vi "5) Target Groups.vi"() -> ()   [LabVIEW 2020, in "VectoScratch.lvlib"]
uses:
  VectoScratch.lvlib
  Vecto/Connection State.ctl
  Vecto/proto/TcpClientHello/Data.ctl
  Simple TCP Handler/Simple TCP Handler.lvclass
  C:/dev/lv20CE/relink/lv-vecto/Vecto/TCPConnectionHandler/TCPConnectionHandler.lvclass
  C:/dev/lv20CE/relink/lv-vecto/Vecto/TCPMessageHandler/TCPMessageHandler.lvclass
  Vecto/TCPMessaging/TCPMessaging.lvclass
  Vecto/TCPMessageService/TCPMessageAPI.lvclass
  Vecto/proto/TcpClientHello/TcpClientHello.lvlib
  Vecto/SequenceCountService/SequenceCountService.lvclass
  Vecto/Vecto.lvlib
panel:
  in  "Stop 3":bool
  in  "Target 3":u32=5
  in  "Target 2":u32=7
  in  "Target 1":u32=6
  in  "Groups":cluster{"Targets":u32[]}[](array[cluster])=[{"Targets"=[4, 5, 7]}, {"Targets"=[4, 5, 6]}, {"Targets"=[4, 6, 7]}]
  in  "Send 3":bool
  out "Read 3":i32
  in  "Send 2":bool
  out "Read 2":i32
  in  "Send 1":bool
  out "Read 1":i32
  out "Error 2":errorcluster
  in  "Stop 2":bool
  out "State 2":T1=enum."Disconnected"
  out "Server Error":errorcluster
  out "Error 1":errorcluster
  in  "Stop 1":bool
  out "State 3":T1=enum."Disconnected"
  out "State 1":T1=enum."Disconnected"
  # "Each node (Clients 1 & 2, Server 3) should also receive data for the targets configured below.\n\nEach row is each of the nodes in order."
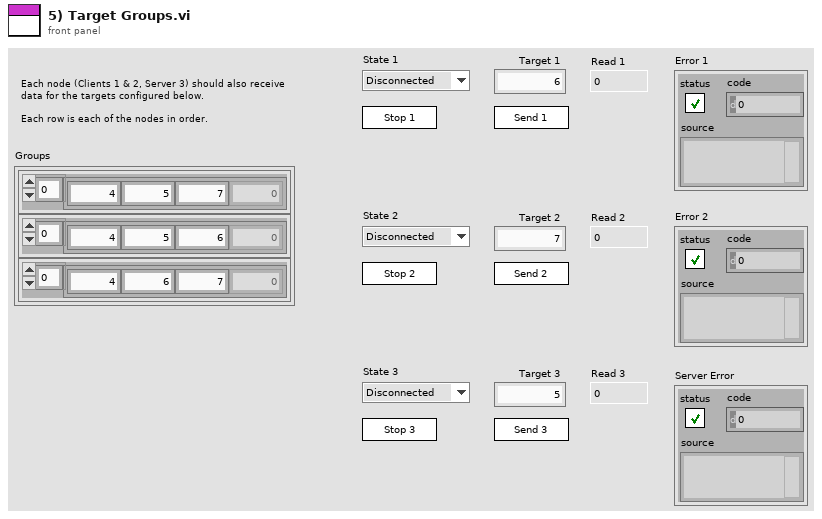
[diagram p1: front panel]
types:
  T1 = typedef "Vecto.lvlib/Connection State.ctl" = enum16{"Connected", "Disconnected"}
  T2 = typedef "TcpClientHello.lvlib/Data.ctl" = cluster{"node_id":u32, "system":string, "cluster":string, "node_name":string, "app_version":string, "config_version":string}
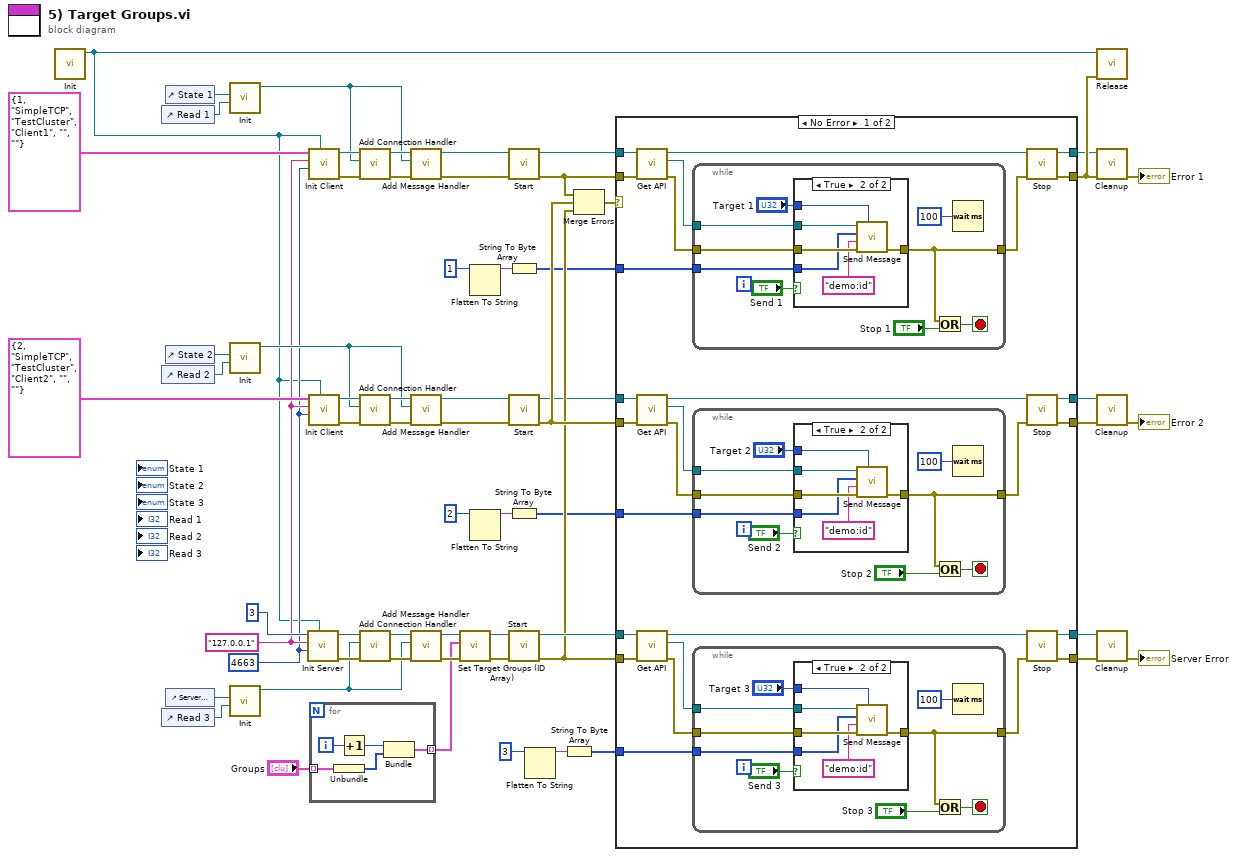
[diagram p0: block diagram]
diagram:
  w2 = u16 4663 ("Bind Port")
  w3 = "127.0.0.1" ("Bind Address")
  n1 = call "Init.vi"() -> ("SequenceCountService out"=w1:refnum<class "SequenceCountService.lvclass">)  [unwired: 10 in, 1 out]
  n2 = control-ref of="Read 1"() -> (w25:refnum<vi>)
  n3 = control-ref of="Read 2"() -> (w24:refnum<vi>)
  n4 = control-ref of="Read 3"() -> (w17:refnum<vi>)
  n5 = control-ref of="State 1"() -> (w59:refnum<vi>)
  n6 = control-ref of="State 2"() -> (w26:refnum<vi>)
  n7 = control-ref of="Server State"() -> (w51:refnum<vi>)
  n8 = call "Init.vi"("Value"=w25, "State"=w59) -> ("Simple TCP Handler out"=w55:refnum<class "Simple TCP Handler.lvclass">)  [unwired: 8 in, 1 out]
  n9 = call "Init.vi"("Value"=w24, "State"=w26) -> ("Simple TCP Handler out"=w23:refnum<class "Simple TCP Handler.lvclass">)  [unwired: 8 in, 1 out]
  n10 = call "Init.vi"("Value"=w17, "State"=w51) -> ("Simple TCP Handler out"=w36:refnum<class "Simple TCP Handler.lvclass">)  [unwired: 8 in, 1 out]
  n11 = call "Init Server.vi"("SequenceCountService"=w1, "Bind Port"=w2, "Bind Address"=w3, "Node ID"=u32 3) -> ("error out"=w46:errorcluster, "TCPMessaging out"=w47:refnum<class "TCPMessaging.lvclass">)  [unwired: 6 in]
  n12 = call "Init Client.vi"("SequenceCountService"=w1, "Remote Port"=w2, "Remote Address"=w3, "Client Info"=T2 {"node_id"=1, "system"="SimpleTCP", "cluster"="TestCluster", "node_name"="Client1", "app_version"="", "config_version"=""}) -> ("error out"=w57:errorcluster, "TCPMessaging out"=w58:refnum<class "TCPMessaging.lvclass">)  [unwired: 6 in]
  n13 = call "Init Client.vi"("SequenceCountService"=w1, "Remote Port"=w2, "Remote Address"=w3, "Client Info"=T2 {"node_id"=2, "system"="SimpleTCP", "cluster"="TestCluster", "node_name"="Client2", "app_version"="", "config_version"=""}) -> ("error out"=w28:errorcluster, "TCPMessaging out"=w27:refnum<class "TCPMessaging.lvclass">)  [unwired: 6 in]
  n14 = for {
    tunnel: "Groups" -> [w66] mode=indexing
    tunnel: [w63] -> w18 mode=indexing
    i -> [w67]
    n15 = Unbundle(w66) -> ("Targets"=w64:u32[])
    n16 = Increment(x=w67) -> (x+1=w65:i32)
    n17 = Bundle(w65, "Targets"=w64) -> (w63:cluster{i32, "Targets":u32[]})  [unwired: 1 in]
  }
  n18 = call "Add Connection Handler.vi"("error in (no error)"=w57, "TCPConnectionHandler"=w55, "TCPMessaging in"=w58) -> ("error out"=w54:errorcluster, "TCPMessaging out"=w56:refnum<class "TCPMessaging.lvclass">)  [unwired: 7 in]
  n19 = call "Add Connection Handler.vi"("error in (no error)"=w28, "TCPConnectionHandler"=w23, "TCPMessaging in"=w27) -> ("error out"=w30:errorcluster, "TCPMessaging out"=w29:refnum<class "TCPMessaging.lvclass">)  [unwired: 7 in]
  n20 = call "Add Connection Handler.vi"("error in (no error)"=w46, "TCPConnectionHandler"=w36, "TCPMessaging in"=w47) -> ("error out"=w49:errorcluster, "TCPMessaging out"=w48:refnum<class "TCPMessaging.lvclass">)  [unwired: 7 in]
  n21 = call "Add Message Handler.vi"("error in (no error)"=w54, "TCPMessageHandler"=w55, "TCPMessaging in"=w56) -> ("error out"=w52:errorcluster, "TCPMessaging out"=w53:refnum<class "TCPMessaging.lvclass">)  [unwired: 7 in]
  n22 = call "Add Message Handler.vi"("error in (no error)"=w30, "TCPMessageHandler"=w23, "TCPMessaging in"=w29) -> ("error out"=w32:errorcluster, "TCPMessaging out"=w31:refnum<class "TCPMessaging.lvclass">)  [unwired: 7 in]
  n23 = call "Add Message Handler.vi"("error in (no error)"=w49, "TCPMessageHandler"=w36, "TCPMessaging in"=w48) -> ("error out"=w50:errorcluster, "TCPMessaging out"=w20:refnum<class "TCPMessaging.lvclass">)  [unwired: 7 in]
  n24 = call "Set Target Groups (ID Array).vi"("error in (no error)"=w50, "Target Groups"=w18, "TCPMessaging in"=w20) -> ("error out"=w21:errorcluster, "TCPMessaging out"=w19:refnum<class "TCPMessaging.lvclass">)  [unwired: 7 in]
  n25 = Flatten To String(anything=1) -> (data string=w12:string)  [unwired: 3 in, 2 out]
  n26 = Flatten To String(anything=2) -> (data string=w7:string)  [unwired: 3 in, 2 out]
  n27 = call "Start.vi"("error in (no error)"=w52, "TCPMessaging in"=w53) -> ("error out"=w44:errorcluster, "TCPMessaging out"=w42:refnum<class "TCPMessaging.lvclass">)  [unwired: 8 in]
  n28 = String To Byte Array(string=w12) -> (unsigned byte array=w10:u8[])
  n29 = call "Start.vi"("error in (no error)"=w32, "TCPMessaging in"=w31) -> ("error out"=w62:errorcluster, "TCPMessaging out"=w16:refnum<class "TCPMessaging.lvclass">)  [unwired: 8 in]
  n30 = String To Byte Array(string=w7) -> (unsigned byte array=w9:u8[])
  n31 = call "Start.vi"("error in (no error)"=w21, "TCPMessaging in"=w19) -> ("error out"=w34:errorcluster, "TCPMessaging out"=w43:refnum<class "TCPMessaging.lvclass">)  [unwired: 8 in]
  n32 = Flatten To String(anything=3) -> (data string=w6:string)  [unwired: 3 in, 2 out]
  n33 = String To Byte Array(string=w6) -> (unsigned byte array=w4:u8[])
  n34 = Merge Errors(w44, w62, w34) -> (w45:errorcluster)
  n35 = case shown="No Error" w45 {
    tunnel: w44 -> [w93 w148]
    tunnel: w34 -> [w91 w147]
    tunnel: w43 -> [w92 w146]
    tunnel: w42 -> [w94 w145]
    tunnel: [w82 w148] -> w61
    tunnel: [w84 w147] -> w39
    tunnel: [w85 w146] -> w40
    tunnel: [w86 w145] -> w41
    tunnel: w16 -> [w76 w144]
    tunnel: w62 -> [w74 w143]
    tunnel: [w80 w144] -> w15
    tunnel: [w79 w143] -> w14
    tunnel: w10 -> [w81 _]
    tunnel: w9 -> [w78 _]
    tunnel: w4 -> [w77 _]
    frame No Error {
      n36 = call "Get API.vi"("error in (no error)"=w93, "TCPMessaging in"=w94) -> ("error out"=w89:errorcluster, "TCP Messaging API"=w90:refnum<class "TCPMessageAPI.lvclass">, "TCPMessaging out"=w87:refnum<class "TCPMessaging.lvclass">)  [unwired: 7 in]
      n37 = call "Get API.vi"("error in (no error)"=w74, "TCPMessaging in"=w76) -> ("error out"=w73:errorcluster, "TCP Messaging API"=w72:refnum<class "TCPMessageAPI.lvclass">, "TCPMessaging out"=w75:refnum<class "TCPMessaging.lvclass">)  [unwired: 7 in]
      n38 = call "Get API.vi"("error in (no error)"=w91, "TCPMessaging in"=w92) -> ("error out"=w71:errorcluster, "TCP Messaging API"=w70:refnum<class "TCPMessageAPI.lvclass">, "TCPMessaging out"=w88:refnum<class "TCPMessaging.lvclass">)  [unwired: 7 in]
      n39 = while {
        tunnel: w90 -> [w119]
        tunnel: w89 -> [w118]
        tunnel: [w114] -> w83
        tunnel: w81 -> [w112]
        stop <- w115 stop-if-true
        n40 = case shown="True" "Send 1" {
          tunnel: w119 -> [_ w126]
          tunnel: w118 -> [w120 w125]
          tunnel: [w120 w124] -> w114
          tunnel: "Target 1" -> [_ w123]
          tunnel: w112 -> [_ w122]
          frame False {
          }
          frame True {
            n41 = call "Send Message.vi"("Target ID"=w123, "error in (no error)"=w125, "Type"="demo:id", "Payload"=w122, "TCPMessageService in"=w126) -> ("error out"=w124:errorcluster)  [unwired: 5 in, 1 out]
          }
        }
        n42 = Or(x=w114, y="Stop 1") -> (x .or. y?=w115:bool)
        n43 = Wait (ms)(milliseconds to wait=u32 100) -> ()  [unwired: 1 out]
      }
      n44 = while {
        tunnel: w72 -> [w103]
        tunnel: w73 -> [w102]
        tunnel: [w99] -> w68
        tunnel: w78 -> [w98]
        stop <- w100 stop-if-true
        n45 = case shown="True" "Send 2" {
          tunnel: w103 -> [_ w110]
          tunnel: w102 -> [w104 w109]
          tunnel: [w104 w108] -> w99
          tunnel: "Target 2" -> [_ w107]
          tunnel: w98 -> [_ w106]
          frame False {
          }
          frame True {
            n46 = call "Send Message.vi"("Target ID"=w107, "error in (no error)"=w109, "Type"="demo:id", "Payload"=w106, "TCPMessageService in"=w110) -> ("error out"=w108:errorcluster)  [unwired: 5 in, 1 out]
          }
        }
        n47 = Or(x=w99, y="Stop 2") -> (x .or. y?=w100:bool)
        n48 = Wait (ms)(milliseconds to wait=u32 100) -> ()  [unwired: 1 out]
      }
      n49 = while {
        tunnel: w70 -> [w135]
        tunnel: w71 -> [w134]
        tunnel: [w131] -> w69
        tunnel: w77 -> [w130]
        stop <- w132 stop-if-true
        n50 = case shown="True" "Send 3" {
          tunnel: w135 -> [_ w142]
          tunnel: w134 -> [w136 w141]
          tunnel: [w136 w140] -> w131
          tunnel: "Target 3" -> [_ w139]
          tunnel: w130 -> [_ w138]
          frame False {
          }
          frame True {
            n51 = call "Send Message.vi"("Target ID"=w139, "error in (no error)"=w141, "Type"="demo:id", "Payload"=w138, "TCPMessageService in"=w142) -> ("error out"=w140:errorcluster)  [unwired: 5 in, 1 out]
          }
        }
        n52 = Or(x=w131, y="Stop 3") -> (x .or. y?=w132:bool)
        n53 = Wait (ms)(milliseconds to wait=u32 100) -> ()  [unwired: 1 out]
      }
      n54 = call "Stop.vi"("error in (no error)"=w83, "TCPMessaging in"=w87) -> ("error out"=w82:errorcluster, "TCPMessaging out"=w86:refnum<class "TCPMessaging.lvclass">)  [unwired: 8 in]
      n55 = call "Stop.vi"("error in (no error)"=w68, "TCPMessaging in"=w75) -> ("error out"=w79:errorcluster, "TCPMessaging out"=w80:refnum<class "TCPMessaging.lvclass">)  [unwired: 8 in]
      n56 = call "Stop.vi"("error in (no error)"=w69, "TCPMessaging in"=w88) -> ("error out"=w84:errorcluster, "TCPMessaging out"=w85:refnum<class "TCPMessaging.lvclass">)  [unwired: 8 in]
    }
    frame Error {
    }
  }
  n57 = call "Release.vi"("error in (no error)"=w61, "SequenceCountService in"=w1) -> ()  [unwired: 9 in, 1 out]
  n58 = call "Cleanup.vi"("error in (no error)"=w61, "TCPMessaging in"=w41) -> ("error out"=→"Error 1":errorcluster)  [unwired: 9 in]
  n59 = call "Cleanup.vi"("error in (no error)"=w14, "TCPMessaging in"=w15) -> ("error out"=→"Error 2":errorcluster)  [unwired: 9 in]
  n60 = call "Cleanup.vi"("error in (no error)"=w39, "TCPMessaging in"=w40) -> ("error out"=→"Server Error":errorcluster)  [unwired: 9 in]
